vi "LoadFromFile.vi"(8 "error in (no error)":errorcluster, 11 "UDP_Config in":refnum<class "UDP_Config.lvclass">) -> (0 "error out":errorcluster, 3 "UDP_Config out":refnum<class "UDP_Config.lvclass">)   [LabVIEW 2021, in "UDP_Config.lvclass"]
uses:
  UDP_Config.lvclass
  UDP_Config.lvclass/UDP_Config.ctl
  <vilib>/Utility/config.llb/NI_LVConfig.lvlib
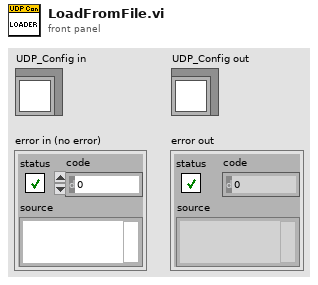
[diagram p1: front panel]
types:
  T1 = typedef "NI_LVConfig.lvlib/Config Data RefNum.ctl" = refnum<k1>
  T2 = typedef "Identity.ctl" = cluster{"NodeID":string, "Role":T3}
  T3 = typedef "Role.ctl" = enum16{"Undefined", "Sender", "Receiver"}
  T4 = typedef "Network.ctl" = cluster{"MulticastGroup":string, "Port":u16, "LocalInterface":string, "TTL":u8}
  T5 = typedef "Diagnostics.ctl" = cluster{"LogEnabled":bool, "LogPath":string}
  T6 = typedef "Sender.ctl" = cluster{"SendIntervalMs":u32, "MaxPayloadBytes":u32}
  T7 = typedef "Receiver.ctl" = cluster{"SocketTimeoutMs":i32, "FilterNodeID":string, "WatchdogTimeoutMs":u32}
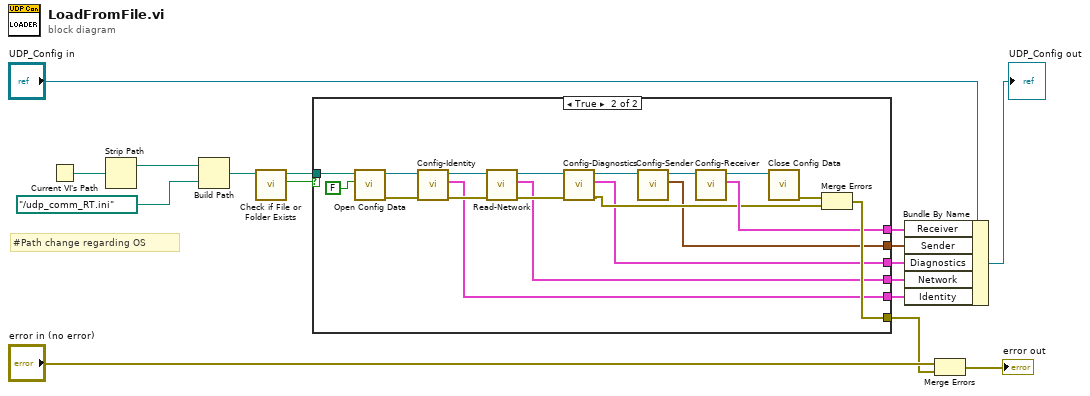
[diagram p0: block diagram]
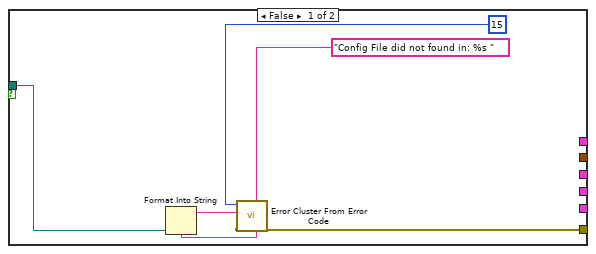
[diagram p2: hidden frame]
diagram:
  # "#Path change regarding OS"
  n1 = Current VI's Path() -> (path=w14:path)
  n2 = Strip Path(path=w14) -> (stripped path=w13:path)  [unwired: 1 out]
  n3 = Build Path(base path=w13, name or relative path=path "../udp_comm_RT.ini" ("path")) -> (appended path=w11:path)
  n4 = call <vilib>:"Check if File or Folder Exists.vi"("path"=w11) -> ("file or folder exists?"=w9:bool, "dup path"=w8:path)  [unwired: 8 in, 1 out]
  n5 = case shown="True" w9 {
    tunnel: w8 -> [w18 w40]
    tunnel: [w21 w33] -> w7
    tunnel: [_ w32] -> w5
    tunnel: [_ w25] -> w4
    tunnel: [_ w24] -> w3
    tunnel: [_ w23] -> w2
    tunnel: [_ w22] -> w1
    frame False {
      n6 = Format Into String(format string="Config File did not found in: %s ", w18) -> (resulting string=w17:string)  [unwired: 2 in, 1 out]
      n7 = call <vilib>:"Error Cluster From Error Code.vi"("error message (\"\")"=w17, "error code (0)"=15) -> ("error out"=w21:errorcluster)  [unwired: 7 in]
    }
    frame True {
      n8 = call <vilib>:"Open Config Data.vi"("create file if necessary (T)"=FALSE, "configuration file path"=w40) -> ("error out"=w37:errorcluster, "refnum"=w38:T1)  [unwired: 7 in, 1 out]
      n9 = call "Config-Identity.vi"("error in"=w37, "Refnum in"=w38) -> ("error out"=w36:errorcluster, "Identity"=w22:T2, "Refnum out"=w35:T1)  [unwired: 7 in]
      n10 = call "Read-Network.vi"("error in (no error)"=w36, "Refnum in"=w35) -> ("error out"=w30:errorcluster, "Network"=w23:T4, "Refnum out"=w31:T1)  [unwired: 7 in]
      n11 = call "Config-Diagnostics.vi"("error in (no error)"=w30, "Refnum in"=w31) -> ("error out"=w27:errorcluster, "Diagnostics"=w24:T5, "Refnum out"=w29:T1)  [unwired: 7 in]
      n12 = call "Config-Sender.vi"("Refnum in"=w29) -> ("Sender"=w25:T6, "Refnum out"=w34:T1)  [unwired: 8 in, 1 out]
      n13 = call "Config-Receiver.vi"("Refnum in"=w34) -> ("Receiver"=w32:T7, "Refnum out"=w28:T1)  [unwired: 8 in, 1 out]
      n14 = call <vilib>:"Close Config Data.vi"("refnum"=w28) -> ("error out"=w26:errorcluster)  [unwired: 9 in, 1 out]
      n15 = Merge Errors(w26, w27) -> (w33:errorcluster)
    }
  }
  n16 = Bundle By Name(cluster="UDP_Config in", "Receiver"=w5, "Sender"=w4, "Diagnostics"=w3, "Network"=w2, "Identity"=w1) -> (→"UDP_Config out":refnum<class "UDP_Config.lvclass">)
  n17 = Merge Errors("error in (no error)", w7) -> (→"error out":errorcluster)
